vi "str to bytestring.vi"(2 "String":string) -> (6 "value":u8[](array[numeric]))   [LabVIEW 2014, in "OPCUA XML.lvlib"]
uses:
  OPCUA XML.lvlib
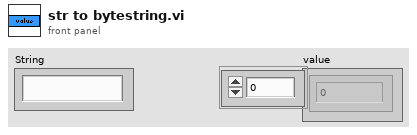
[diagram p1: front panel]
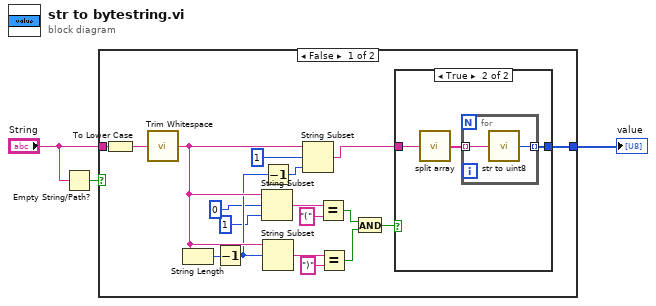
[diagram p0: block diagram]
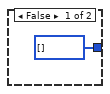
[diagram p2: hidden frame]
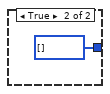
[diagram p3: hidden frame]
diagram:
  n1 = Empty String/Path?(string/path="String") -> (empty?=w1:bool)
  n2 = case shown="False" w1 {
    tunnel: [w20 u8[] []] -> w3
    tunnel: "String" -> [w18 _]
    frame False {
      n3 = To Lower Case(string=w18) -> (all lower case string=w21:string)
      n4 = call <vilib>:"Trim Whitespace.vi"("string"=w21) -> ("trimmed string"=w10:string)  [unwired: 1 in]
      n5 = String Length(string=w10) -> (length=w19:i32)
      n6 = Decrement(x=w19) -> (x-1=w6:i32)
      n7 = String Subset(string=w10, offset (0)=0 ("length (rest)"), length (rest)=1 ("length (rest)")) -> (substring=w17:string)
      n8 = Decrement(x=w6) -> (x-1=w7:i32)
      n9 = String Subset(string=w10, offset (0)=w6) -> (substring=w16:string)  [unwired: 1 in]
      n10 = String Subset(string=w10, offset (0)=1 ("length (rest)"), length (rest)=w7) -> (substring=w9:string)
      n11 = Equal?(x=w17, y="(") -> (x = y?=w13:bool)
      n12 = Equal?(x=w16, y=")") -> (x = y?=w12:bool)
      n13 = And(x=w13, y=w12) -> (x .and. y?=w11:bool)
      n14 = case shown="True" w11 {
        tunnel: [u8[] [] w24] -> w20
        tunnel: w9 -> [_ w23]
        frame False {
        }
        frame True {
          n15 = call "split array.vi"("string"=w23) -> ("split arr"=w25:string[])  [unwired: 8 in]
          n16 = for {
            tunnel: w25 -> [w27] mode=indexing
            tunnel: [w26] -> w24 mode=indexing
            n17 = call "str to uint8.vi"("String"=w27) -> ("uint8"=w26:u8)  [unwired: 6 in]
          }
        }
      }
    }
    frame True {
    }
  }
  "value" <- w3
